vi "Clear Buffers.vi"(8 "error in (no error)":errorcluster, 11 "Readable in":refnum<class "Readable.lvclass">) -> (0 "error out":errorcluster, 3 "Readable out":refnum<class "Readable.lvclass">)   [LabVIEW 2015, in "Readable.lvclass"]
uses:
  Readable.lvclass
  Readable.lvclass/Readable.ctl
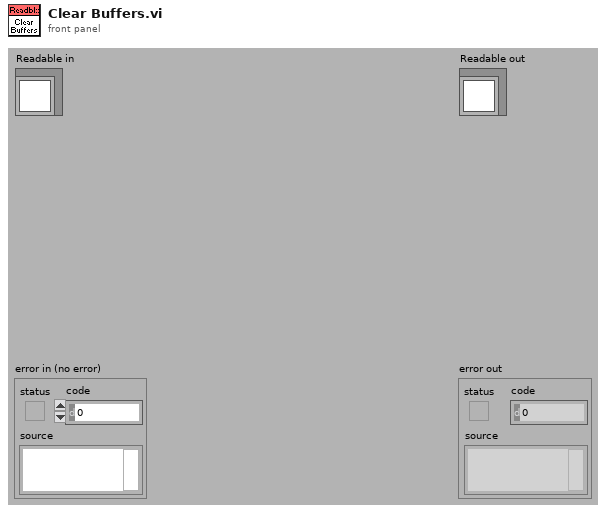
[diagram p1: front panel]
types:
  T1 = cluster{"Data Points":cluster{"t":timestamp, "x":dbl}[]}
  T2 = typedef "Readable.lvclass/Channel Names.ctl" = string[]
  T3 = cluster{"Data Points":cluster{"t":timestamp, "x":dbl}[]}[]
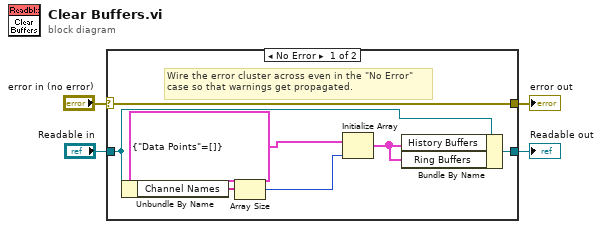
[diagram p0: block diagram]
diagram:
  n1 = case shown="No Error" "error in (no error)" {
    selector: "error in (no error)" -> [w11 w13]
    tunnel: [w11 w13] -> w3
    tunnel: [w10 w12] -> w1
    tunnel: "Readable in" -> [w9 w12]
    frame No Error {
      # "Wire the error cluster across even in the \"No Error\"\ncase so that warnings get propagated."
      n2 = Unbundle By Name(w9) -> ("Channel Names"=w8:T2)
      n3 = Array Size(array=w8) -> (size(s)=w7:i32)
      n4 = Initialize Array(T1 {"Data Points"=[]}, w7) -> (w6:T3)
      n5 = Bundle By Name(cluster=w9, "History Buffers"=w6, "Ring Buffers"=w6) -> (w10:refnum<class "Readable.lvclass">)
    }
    frame Error {
    }
  }
  "error out" <- w3
  "Readable out" <- w1
